vi "Show Bookmark.vi"(8 "Error In":errorcluster, 10 "Bookmarks":T1[](array[typedef]), 11 "Tag":string) -> (0 "Error Out":errorcluster)   [LabVIEW 2018, in "Bookmark Manager.lvlib"]
uses:
  Bookmark Manager.lvlib
  Controls/Bookmark.ctl
  Controls/VI Identifier.ctl
  <vilib>/addons/analyzer/_analyzerctrls.llb/VIAnCtl Analysis App Info.ctl
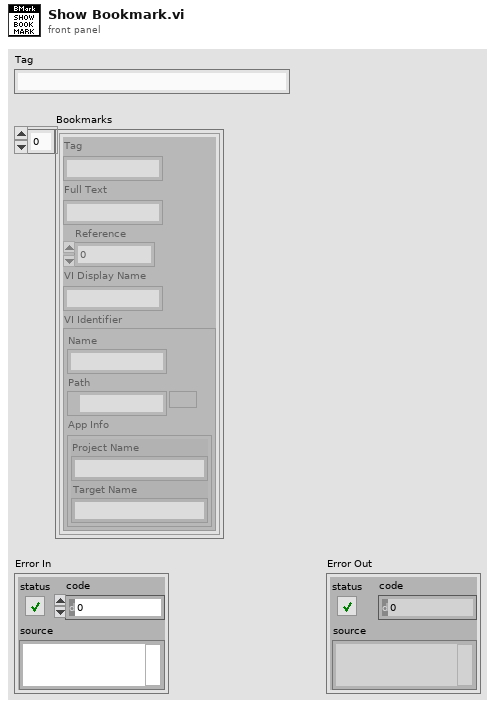
[diagram p1: front panel]
types:
  T1 = typedef "Bookmark Manager.lvlib/Bookmark.ctl" = cluster{"Tag":string, "Full Text":string, "Reference":i32, "VI Display Name":string, "VI Identifier":T2}
  T2 = typedef "Bookmark Manager.lvlib/VI Identifier.ctl" = cluster{"Name":string, "Path":path, "App Info":T3}
  T3 = typedef "VIAnCtl Analysis App Info.ctl" = cluster{"Project Name":string, "Target Name":string}
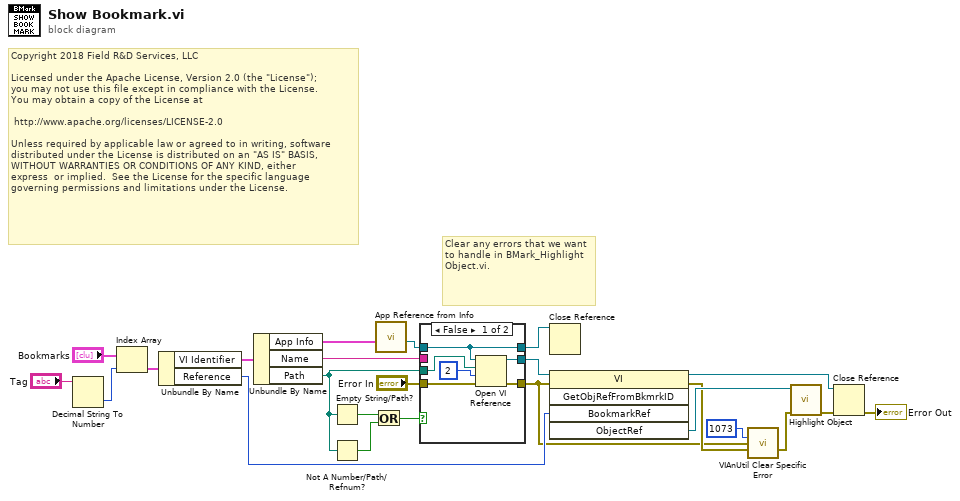
[diagram p0: block diagram]
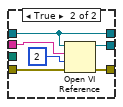
[diagram p2: hidden frame]
diagram:
  # "Copyright 2018 Field R&D Services, LLC\n\nLicensed under the Apache License, Version 2.0 (the \"License\");\nyou may not use this file except in compliance with the License.\nYou may obtain a copy of the License at\n\n\thttp://www.apache.org/licenses/LICENSE-2.0\n\nUnless required by applicable law or agreed to in writing, software\ndistributed under the License is distributed on an \"AS IS\" BASIS,\nWITHOUT WARRANTIES OR CONDITIONS OF ANY KIND, either \nexpress  or implied.  See the License for the specific language \ngoverning permissions and limitations under the License."
  # "Clear any errors that we want to handle in BMark_Highlight Object.vi."
  n1 = Decimal String To Number(string="Tag") -> (number=w22:i32)  [unwired: 2 in, 1 out]
  n2 = Index Array(array="Bookmarks", index=w22) -> (element=w21:T1)
  n3 = Unbundle By Name(w21) -> ("VI Identifier"=w20:T2, "Reference"=w16:i32)
  n4 = Unbundle By Name(w20) -> ("App Info"=w10:T3, "Name"=w19:string, "Path"=w8:path)
  n5 = Empty String/Path?(string/path=w8) -> (empty?=w7:bool)
  n6 = Not A Number/Path/Refnum?(number/path/refnum=w8) -> (NaN/Path/Refnum?=w6:bool)
  n7 = Or(x=w7, y=w6) -> (x .or. y?=w5:bool)
  n8 = call "App Reference from Info.vi"("Analysis App Info"=w10) -> ("Analysis App Ref"=w9:refnum<vi>)  [unwired: 9 in, 1 out]
  n9 = case shown="False" w5 {
    tunnel: w19 -> [_ w36]
    tunnel: w9 -> [w25 w31]
    tunnel: [w30 w35] -> w17
    tunnel: w8 -> [w29 _]
    tunnel: "Error In" -> [w28 w34]
    tunnel: [w27 w33] -> w1
    tunnel: [w25 w31] -> w11
    frame False {
      n10 = Open VI Reference(application reference (local)=w25, vi path=w29, options=2, error in (no error)=w28) -> (vi reference=w30:refnum<vi>, error out=w27:errorcluster)  [unwired: 2 in]
    }
    frame True {
      n11 = Open VI Reference(application reference (local)=w31, vi path=w36, options=2, error in (no error)=w34) -> (vi reference=w35:refnum<vi>, error out=w33:errorcluster)  [unwired: 2 in]
    }
  }
  n12 = Close Reference(reference=w11) -> ()  [unwired: 1 in, 1 out]
  n13 = invoke class="VI" method="GetObjRefFromBkmrkID"(reference=w17, error in=w1, "BookmarkRef"=w16) -> (reference out=w12:refnum<vi>, error out=w4:errorcluster, "ObjectRef"=w15:refnum<vi>)  [unwired: 2 in, 2 out]
  n14 = call <vilib>:"VIAnUtil Clear Specific Error.vi"("Error of Interest"=1073, "error in (previous)"=w1, "error in (current)"=w4) -> ("error out"=w3:errorcluster)  [unwired: 12 out]
  n15 = call "Highlight Object.vi"("Error In"=w3, "GObj Refnum"=w15) -> ("Error Out"=w14:errorcluster)  [unwired: 9 in]
  n16 = Close Reference(reference=w12, error in (no error)=w14) -> (error out=→"Error Out":errorcluster)
